vi "set_destination.vi"(8 "error in (no error)":errorcluster, 10 "destination":string, 11 "MoAgSy_Engine.lvclass in":refnum<class "MoAgSy_Engine.lvclass">) -> (0 "error out":errorcluster, 3 "MoAgSy_Engine.lvclass out":refnum<class "MoAgSy_Engine.lvclass">)   [LabVIEW 2009, in "MoAgSy.lvlib" / "MoAgSy_Engine.lvclass"]
uses:
  MoAgSy_Engine.lvclass
  MoAgSy_Engine.lvclass/MoAgSy_Engine.ctl
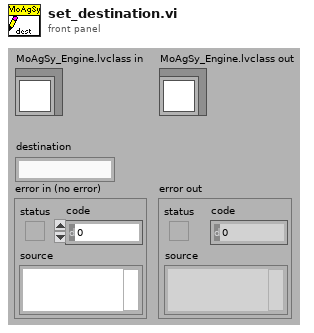
[diagram p1: front panel]
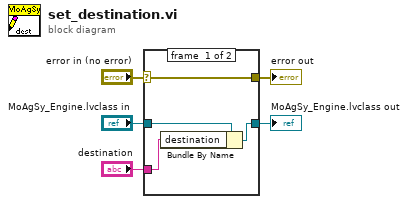
[diagram p0: block diagram]
diagram:
  n1 = case shown="No Error" "error in (no error)" {
    selector: "error in (no error)" -> [w9 w10]
    tunnel: [w9 w10] -> w4
    tunnel: [w7 w11] -> w2
    tunnel: "MoAgSy_Engine.lvclass in" -> [w8 w11]
    tunnel: "destination" -> [w6 _]
    frame #0 {
      n2 = Bundle By Name(cluster=w8, "destination"=w6) -> (w7:refnum<class "MoAgSy_Engine.lvclass">)
    }
    frame #1 {
    }
  }
  "error out" <- w4
  "MoAgSy_Engine.lvclass out" <- w2
